vi "sumArrayElements.vi"() -> ()   [LabVIEW 2024]
panel:
  out "sum":dbl[](array[numeric])
  in  "in":dbl[][](array[numeric])
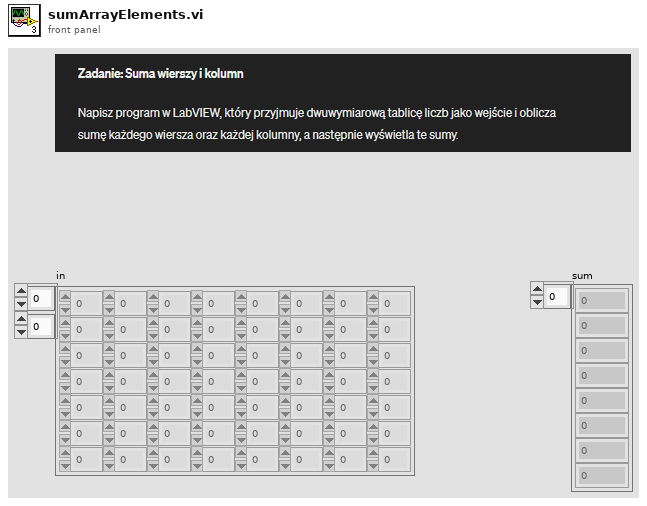
[diagram p1: front panel]
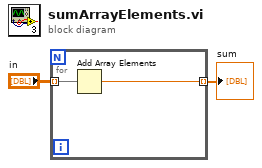
[diagram p0: block diagram]
diagram:
  n1 = for {
    tunnel: "in" -> [w4] mode=indexing
    tunnel: [w3] -> w1 mode=indexing
    n2 = Add Array Elements(numeric array=w4) -> (sum=w3:dbl)
  }
  "sum" <- w1
